vi "Master Manufacturer List.vi"(7 "VISA resource name":refnum<visa-resource-name>, 8 "error in":errorcluster, 9 "Serial":string, 10 "Model":string, 11 "Manufacturer":string) -> (0 "error out":errorcluster, 3 "Generic Instrument out":refnum<class "Generic Instrument.lvclass">)   [LabVIEW 2014, in "SetUp VIs.lvlib"]
uses:
  SetUp VIs.lvlib
  Generic Instrument/Generic Instrument.lvclass
  Universal Power Meter/Universal Power Meter class/Identification/Manufacturer List.ctl
  Universal Power Meter/Universal Power Meter class/Models.ctl
  <vilib>/Utility/error.llb/whitespace.ctl
  Generic Power Analyzer/Tektronix PA1000/Tektronix PA1000.lvclass
  Generic Digital Multi Meter/Tektronix DMM4020/Tektronix DMM4020.lvclass
  Generic Data Acquisition/Fluke Hydra/Fluke Hydra 2625A.lvclass
  Generic Data Acquisition/National Instrument USB-6501/National Instrument USB-6501.lvclass
  Generic Power Analyzer/Yokogawa WT2X0/Yokogawa WT2X0.lvclass
  Generic Power Analyzer/Yokogawa WT500/Yokogawa WT500.lvclass
  Generic Power Analyzer/Yokogawa WT1600/Yokogawa WT1600.lvclass
  Generic Instrument/Generic Instrument.lvclass/Generic Instrument.ctl
  Abstract Sensor/Abstract Sensor.lvclass
panel:
  out "Model Lower":string
  out "list lower":string[](array[string])
  out "index of element":i32
  in  "Model":T1
  in  "Manufacturer Enum":T2=enum."FLUKE"
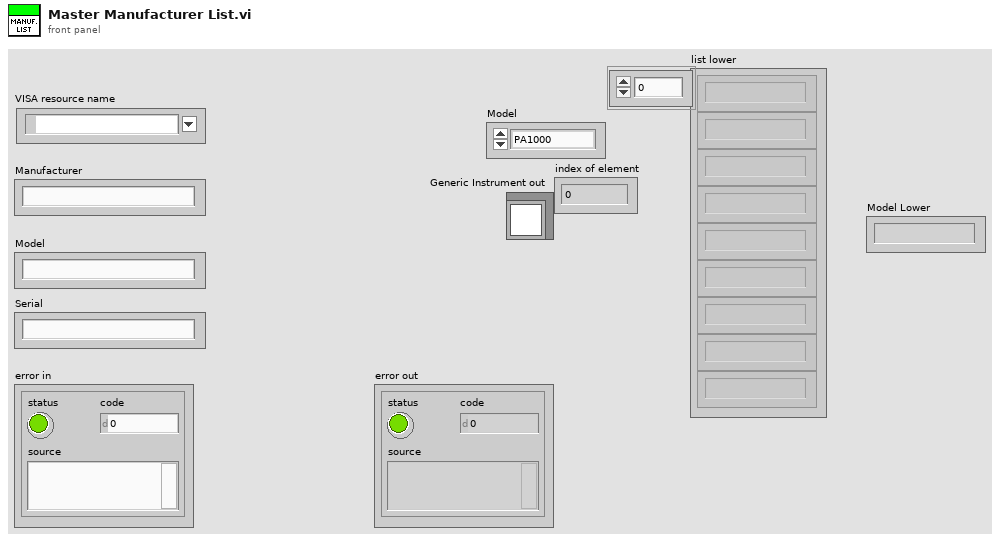
[diagram p1: front panel]
types:
  T1 = typedef "Models.ctl" = enum16{"PA1000", "USB-6501", "2635A", "2625A", "WT500", "WT1600", "DMM4020", "WT230", "WT210"}
  T2 = typedef "Manufacturer List.ctl" = enum16{"NATIONAL INSTRUMENTS", "TEKTRONIX", "FLUKE", "dummy", "red", "YOKOGAWA"}
  T3 = typedef "whitespace.ctl" = u16
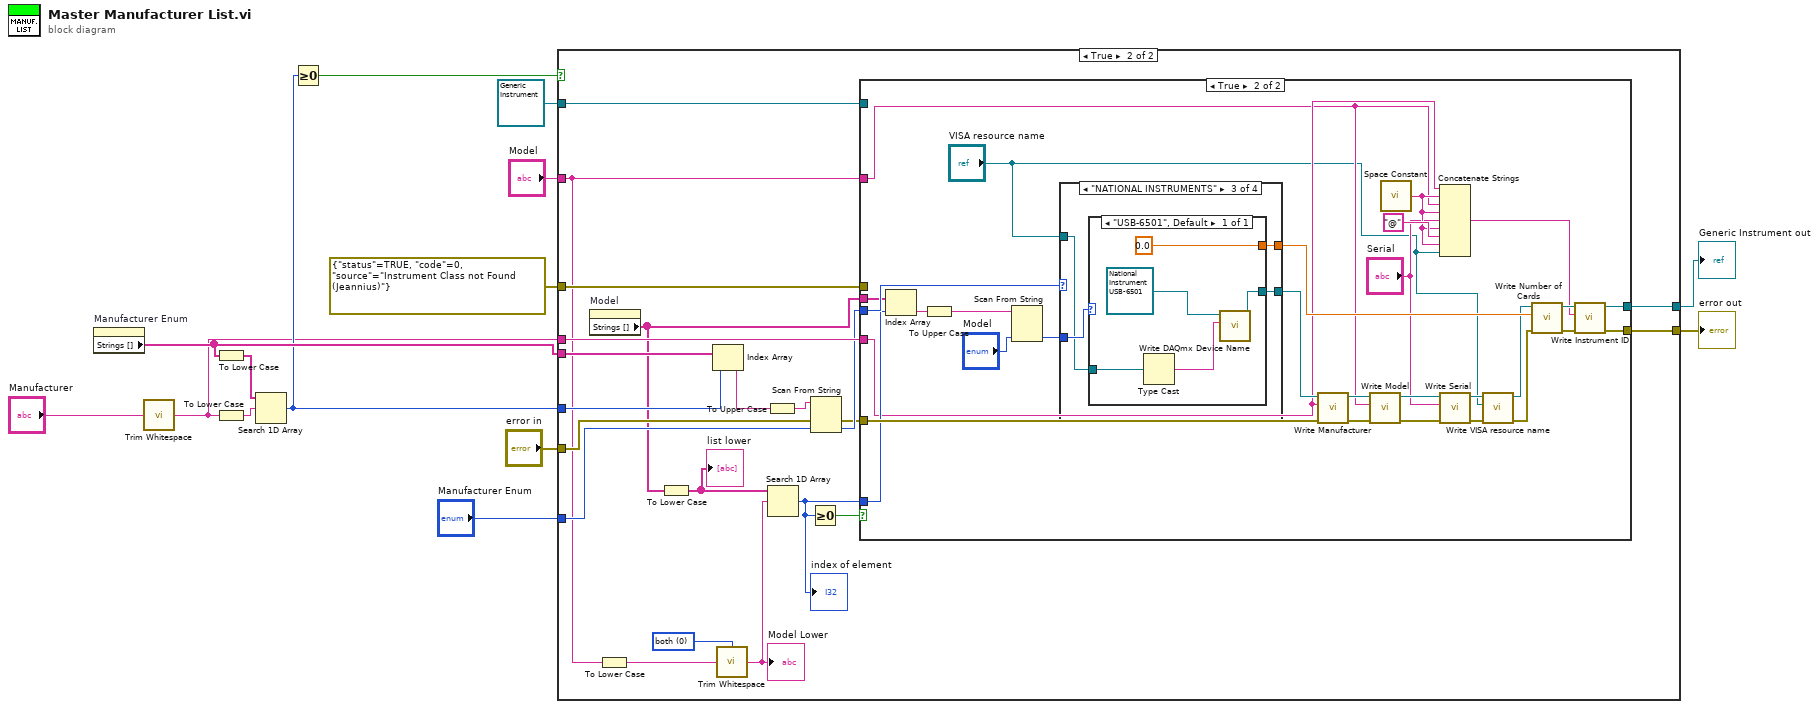
[diagram p0: block diagram]
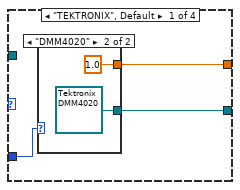
[diagram p4: hidden frame]
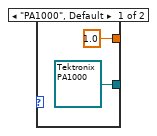
[diagram p5: hidden frame]
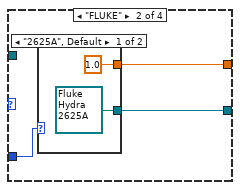
[diagram p6: hidden frame]
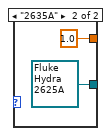
[diagram p7: hidden frame]
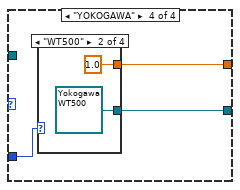
[diagram p8: hidden frame]
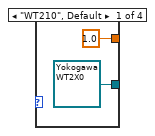
[diagram p9: hidden frame]
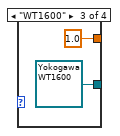
[diagram p10: hidden frame]
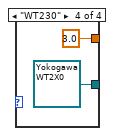
[diagram p11: hidden frame]
diagram:
  n1 = property on="Manufacturer Enum" class="Enum (strict)"() -> ("Strings []"=w9:string[])  [unwired: 2 in, 2 out]
  n2 = call <vilib>:"Trim Whitespace.vi"("string"="Manufacturer") -> ("trimmed string"=w2:string)  [unwired: 1 in]
  n3 = To Lower Case(string=w9) -> (all lower case string=w11:string[])
  n4 = To Lower Case(string=w2) -> (all lower case string=w12:string)
  n5 = Search 1D Array(1D array=w11, element=w12) -> (index of element=w8:i32)  [unwired: 1 in]
  n6 = Greater Or Equal To 0?(x=w8) -> (x >= 0?=w10:bool)
  n7 = case shown="True" w10 {
    tunnel: [w16 w37] -> w14
    tunnel: [w15 w36] -> w13
    tunnel: w2 -> [_ w35]
    tunnel: w9 -> [_ w34]
    tunnel: w8 -> [_ w33]
    tunnel: "Manufacturer Enum" -> [_ w32]
    tunnel: "error in" -> [_ w30]
    tunnel: errorcluster {"status"=TRUE, "code"=0, "source"="Instrument Class not Found (Jeannius)"} ("error out") -> [w16 w24]
    tunnel: refnum<class "Generic Instrument.lvclass"> refnum ("Generic Instrument out") -> [w15 w23]
    tunnel: "Model" -> [_ w17]
    frame False {
    }
    frame True {
      w20 = T3 0 items=["both", "start of string", "end of string"] ("location (both)")
      n8 = property on="Model" class="Enum (strict)"() -> ("Strings []"=w21:string[])  [unwired: 2 in, 2 out]
      n9 = To Lower Case(string=w17) -> (all lower case string=w19:string)
      n10 = To Lower Case(string=w21) -> (all lower case string=w26:string[])
      "list lower" <- w26
      n11 = Index Array(array=w34, index=w33) -> (element=w29:string)
      n12 = call <vilib>:"Trim Whitespace.vi"("string"=w19, "location (both)"=w20) -> ("trimmed string"=w18:string)
      "Model Lower" <- w18
      n13 = To Upper Case(1:w29) -> (0:w28:string)
      n14 = Search 1D Array(1D array=w26, element=w18) -> (index of element=w22:i32)  [unwired: 1 in]
      "index of element" <- w22
      n15 = Greater Or Equal To 0?(x=w22) -> (x >= 0?=w25:bool)
      n16 = Scan From String(input string=w28, error in=w30, default 1=w32) -> (error out=w27:errorcluster, output 1=w31:T2)  [unwired: 2 in, 2 out]
      n17 = case shown="True" w25 {
        tunnel: [w39 w45] -> w37
        tunnel: [w38 w46] -> w36
        tunnel: w35 -> [_ w52]
        tunnel: w31 -> [_ w64]
        tunnel: w27 -> [_ w62]
        tunnel: w17 -> [_ w51]
        tunnel: w24 -> [w39 _]
        tunnel: w23 -> [w38 _]
        tunnel: w22 -> [_ w61]
        tunnel: w21 -> [_ w60]
        frame False {
        }
        frame True {
          n18 = Index Array(array=w60, index=w61) -> (element=w57:string)
          n19 = To Upper Case(1:w57) -> (0:w56:string)
          n20 = Scan From String(input string=w56, default 1="Model") -> (output 1=w58:T1)  [unwired: 3 in, 3 out]
          n21 = case shown="\"NATIONAL INSTRUMENTS\"" w64 {
            tunnel: [w71 w78 w85 w94] -> w63
            tunnel: w58 -> [w70 w77 w86 w93]
            tunnel: [w69 w76 w84 w92] -> w55
            tunnel: "VISA resource name" -> [_ _ w83 _]
            frame "TEKTRONIX", Default {
              n22 = case shown="\"DMM4020\"" w70 {
                tunnel: [refnum<class "Tektronix PA1000.lvclass"> refnum ("Generic Power Analyzer.lvlib:Tektronix PA1000.lvlib:Tektronix PA1000.lvclass") refnum<class "Tektronix DMM4020.lvclass"> refnum ("Generic Digital Multi Meter.lvlib:Tektronix DMM4020.lvlib:Tektronix DMM4020.lvclass")] -> w71
                tunnel: [1.0 1.0] -> w69
                frame "PA1000", Default {
                }
                frame "DMM4020" {
                }
              }
            }
            frame "FLUKE" {
              n23 = case shown="\"2625A\", Default" w77 {
                tunnel: [refnum<class "Fluke Hydra 2625A.lvclass"> refnum ("Generic Data Acquisition.lvlib:Fluke Hydra.lvlib:Fluke Hydra 2625A.lvclass") refnum<class "Fluke Hydra 2625A.lvclass"> refnum ("Generic Data Acquisition.lvlib:Fluke Hydra.lvlib:Fluke Hydra 2625A.lvclass")] -> w78
                tunnel: [1.0 1.0] -> w76
                frame "2625A", Default {
                }
                frame "2635A" {
                }
              }
            }
            frame "NATIONAL INSTRUMENTS" {
              n24 = case shown="\"USB-6501\", Default" w86 {
                tunnel: [w89] -> w85
                tunnel: [0.0] -> w84
                tunnel: w83 -> [w88]
                frame "USB-6501", Default {
                  n25 = Type Cast(x=w88) -> (*(type *) &x=w87:string)  [unwired: 1 in]
                  n26 = call-dynamic "Write DAQmx Device Name.vi"("DAQmx Device Name"=w87, "National Instrument USB-6501 in"=refnum<class "National Instrument USB-6501.lvclass"> refnum ("Generic Data Acquisition.lvlib:National Instrument USB-6501.lvlib:National Instrument USB-6501.lvclass")) -> ("National Instrument USB-6501 out"=w89:refnum<class "National Instrument USB-6501.lvclass">)  [unwired: 8 in, 1 out]
                }
              }
            }
            frame "YOKOGAWA" {
              n27 = case shown="\"WT500\"" w93 {
                tunnel: [refnum<class "Yokogawa WT2X0.lvclass"> refnum ("Generic Power Analyzer.lvlib:Yokogawa WT2X0.lvlib:Yokogawa WT2X0.lvclass") refnum<class "Yokogawa WT500.lvclass"> refnum ("Generic Power Analyzer.lvlib:Yokogawa WT500.lvlib:Yokogawa WT500.lvclass") refnum<class "Yokogawa WT1600.lvclass"> refnum ("Generic Power Analyzer.lvlib:Yokogawa WT1600.lvlib:Yokogawa WT1600.lvclass") refnum<class "Yokogawa WT2X0.lvclass"> refnum ("Generic Power Analyzer.lvlib:Yokogawa WT2X0.lvlib:Yokogawa WT2X0.lvclass")] -> w94
                tunnel: [1.0 1.0 1.0 3.0] -> w92
                frame "WT210", Default {
                }
                frame "WT500" {
                }
                frame "WT1600" {
                }
                frame "WT230" {
                }
              }
            }
          }
          n28 = call "Write Manufacturer.vi"("error in (no error)"=w62, "Manufacturer"=w52, "Generic Instrument in"=w63) -> ("error out"=w66:errorcluster, "Generic Instrument out"=w68:refnum<class "Abstract Sensor.lvclass">)  [unwired: 7 in]
          n29 = call "Write Model.vi"("error in (no error)"=w66, "Model"=w51, "Generic Instrument in"=w68) -> ("error out"=w65:errorcluster, "Generic Instrument out"=w67:refnum<class "Abstract Sensor.lvclass">)  [unwired: 7 in]
          n30 = call <vilib>:"Space Constant.vi"() -> ("String"=w53:string)
          n31 = Concatenate Strings(w52, w53, w51, w53, "Serial", w53, "@", w53, "VISA resource name") -> (w48:string)
          n32 = call-dynamic "Write Serial.vi"("error in (no error)"=w65, "Serial"="Serial", "Generic Instrument in"=w67) -> ("error out"=w43:errorcluster, "Generic Instrument out"=w44:refnum<class "Abstract Sensor.lvclass">)  [unwired: 7 in]
          n33 = call-dynamic "Write VISA resource name.vi"("error in (no error)"=w43, "VISA resource name"="VISA resource name", "Generic Instrument in"=w44) -> ("error out"=w42:errorcluster, "Generic Instrument out"=w41:refnum<class "Abstract Sensor.lvclass">)  [unwired: 7 in]
          n34 = call-dynamic "Write Number of Cards.vi"("error in (no error)"=w42, "Number of Cards"=w55, "Generic Instrument in"=w41) -> ("error out"=w47:errorcluster, "Generic Instrument out"=w49:refnum<class "Abstract Sensor.lvclass">)  [unwired: 7 in]
          n35 = call-dynamic "Write Instrument ID.vi"("error in (no error)"=w47, "Instrument ID"=w48, "Generic Instrument in"=w49) -> ("error out"=w45:errorcluster, "Generic Instrument out"=w46:refnum<class "Abstract Sensor.lvclass">)  [unwired: 7 in]
        }
      }
    }
  }
  "error out" <- w14
  "Generic Instrument out" <- w13
